vi "Get CaseFrame Reference By CaseName.vi"(8 "error in (no error)":errorcluster, 10 "CASE":string, 11 "CSM-Helper in":refnum<class "CSM-Helper.lvclass">) -> (0 "error out":errorcluster, 1 "Frame Refs":refnum<vi>, 3 "CSM-Helper out":refnum<class "CSM-Helper.lvclass">)   [LabVIEW 2017, in "CSM-Helper.lvclass"]
doc: "### Get CaseFrame Reference By CaseName.vi\n\n-- <b>Controls</b> --\n- <b>CASE</b>:\n- <b>CSM-Helper in</b>: CSMHelper input\n\n-- <b>Indicators</b> --\n- <b>Frame Refs</b>:\n- <b>CSM-Helper out</b>: CSMHelper output"
uses:
  CSM-Helper.lvclass
  CSM-Helper.lvclass/CSM-Helper.ctl
  _Shared/CSM Shared.lvlib
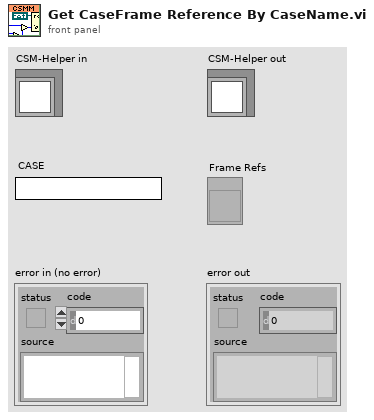
[diagram p1: front panel]
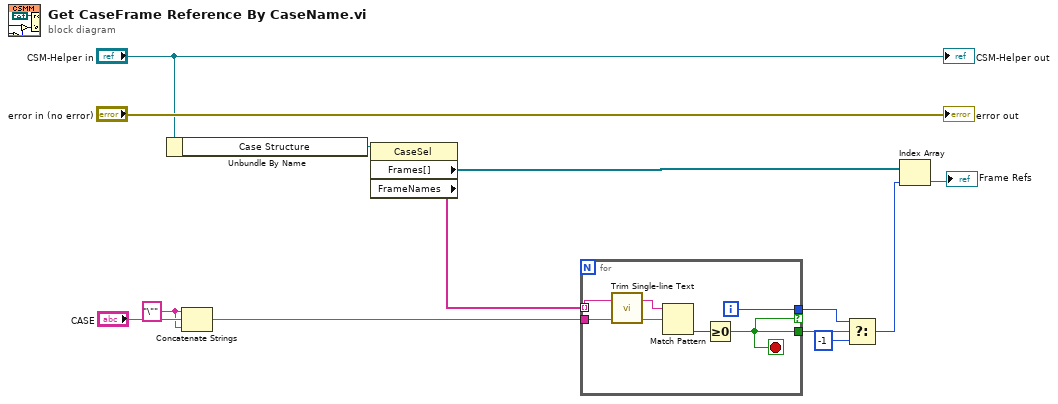
[diagram p0: block diagram]
diagram:
  w7 = "\"" ("string")
  n1 = Unbundle By Name("CSM-Helper in") -> ("Case Structure"=w11:refnum<vi>)
  n2 = Concatenate Strings(w7, "CASE", w7) -> (w8:string)
  n3 = property class="CaseSel"(reference=w11) -> ("Frames[]"=w6:refnum<vi>[], "FrameNames"=w10:string[])  [unwired: 1 in, 2 out]
  n4 = for {
    tunnel: w10 -> [w19] mode=indexing
    tunnel: w8 -> [w18]
    tunnel: [w17] -> w2 if=w15
    tunnel: [w15] -> w4
    i -> [w17]
    stop <- w15 stop-if-true
    n5 = call "Trim Single-line Text.vi"("single-line text"=w19) -> ("trimed text"=w14:string)  [unwired: 2 in]
    n6 = Match Pattern(string=w14, regular expression=w18) -> (offset past match=w16:i32)  [unwired: 1 in, 3 out]
    n7 = Greater Or Equal To 0?(x=w16) -> (x >= 0?=w15:bool)
  }
  n8 = Select(t=w2, s=w4, f=-1) -> (s? t:f=w1:i32)
  n9 = Index Array(array=w6, index=w1) -> (element=→"Frame Refs":refnum<vi>)
  "error out" <- "error in (no error)"
  "CSM-Helper out" <- "CSM-Helper in"
